vi "plant_structure.vi"(9 "Dataflow":errorcluster, 10 "Pause":refnum<vi>, 11 "Stop":refnum<vi>) -> ()   [LabVIEW 2019]
uses:
  lib/libSimulationControl/libSimulationControl.lvlib
panel:
  # "*******************************************************************\nBiogas Plant Control\n\nAuthor: Paul Zügel\nGCSC-Frankfurt am Main 2020\n\n*******************************************************************"
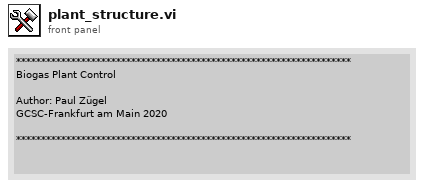
[diagram p1: front panel]
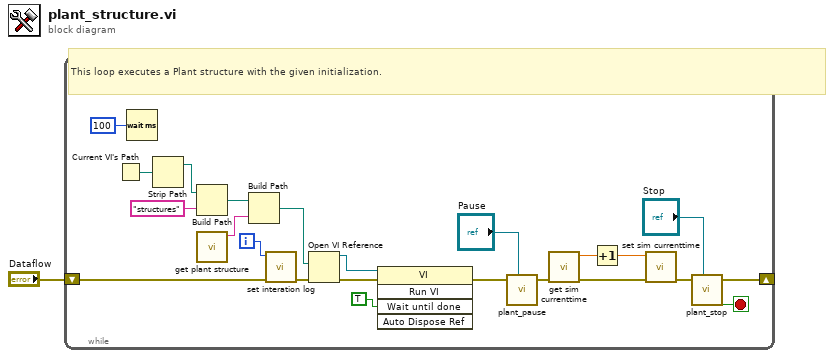
[diagram p0: block diagram]
diagram:
  n1 = while {
    shift-right: [w21] -> _
    shift-left: "Dataflow" -> [w4]
    i -> [w20]
    stop <- w9 stop-if-true
    # "This loop executes a Plant structure with the given initialization."
    n2 = Current VI's Path() -> (path=w18:path)
    n3 = Wait (ms)(milliseconds to wait=u32 100) -> ()  [unwired: 1 out]
    n4 = Strip Path(path=w18) -> (stripped path=w17:path)  [unwired: 1 out]
    n5 = Build Path(base path=w17, name or relative path="structures") -> (appended path=w15:path)
    n6 = call "get plant structure.vi"() -> ("function return"=w19:string)  [unwired: 10 in, 1 out]
    n7 = Build Path(base path=w15, name or relative path=w19) -> (appended path=w14:path)
    n8 = call "set interation log.vi"("error in (no error)"=w4, "iter"=w20) -> ("error out"=w3:errorcluster)  [unwired: 9 in]
    n9 = Open VI Reference(vi path=w14, error in (no error)=w3) -> (vi reference=w10:refnum<vi>, error out=w13:errorcluster)  [unwired: 4 in]
    n10 = invoke class="VI" method="Run VI"(reference=w10, error in=w13, "Wait until done"=TRUE ("Wait Until Done")) -> (error out=w12:errorcluster)  [unwired: 2 in, 4 out]
    n11 = call "plant_pause.vi"("Dataflow In"=w12, "Pause"="Pause") -> ("Dataflow Out"=w6:errorcluster)  [unwired: 5 in]
    n12 = call "get sim currenttime.vi"("error in (no error)"=w6) -> ("error out"=w8:errorcluster, "function return"=w2:dbl)  [unwired: 9 in]
    n13 = Increment(x=w2) -> (x+1=w7:dbl)
    n14 = call "set sim currenttime.vi"("error in (no error)"=w8, "time"=w7) -> ("error out"=w5:errorcluster)  [unwired: 9 in]
    n15 = call "plant_stop.vi"("Dataflow In"=w5, "Stop In"="Stop") -> ("Stop Out"=w9:bool, "Dataflow Out"=w21:errorcluster)  [unwired: 4 in]
  }
